vi "run.vi"(8 "error in (no error)":errorcluster, 11 "AutoExp in":refnum<class "AutoExp.lvclass">) -> (0 "error out":errorcluster, 3 "AutoExp out":refnum<class "AutoExp.lvclass">)   [LabVIEW 2018, in "AutoExp.lvclass"]
uses:
  AutoExp.lvclass
  AutoExp.lvclass/AutoExp.ctl
  State Machine/State Machine.lvclass
  Channel/Channel.lvclass
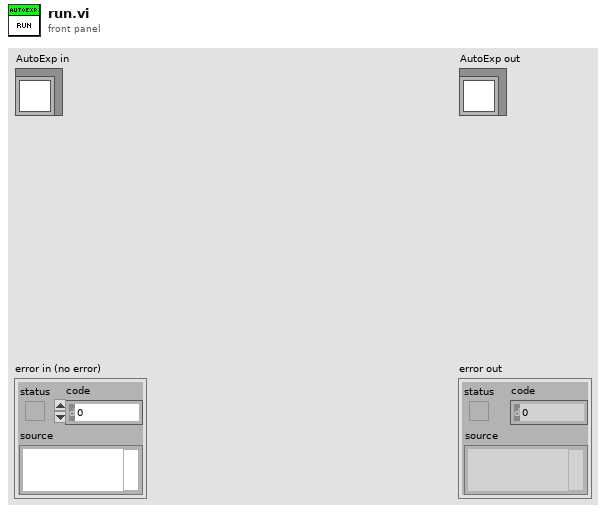
[diagram p1: front panel]
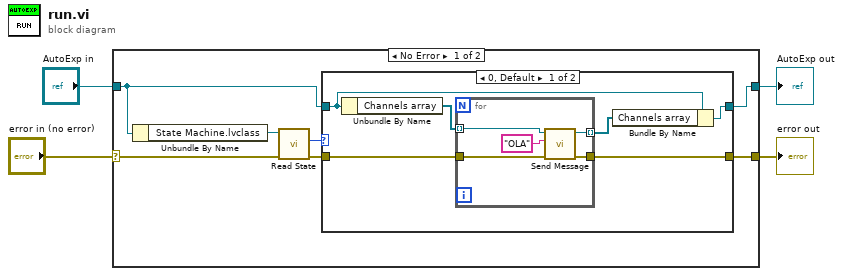
[diagram p0: block diagram]
diagram:
  n1 = case shown="No Error" "error in (no error)" {
    selector: "error in (no error)" -> [w11 w26]
    tunnel: [w7 w26] -> w3
    tunnel: [w5 w25] -> w1
    tunnel: "AutoExp in" -> [w6 w25]
    frame No Error {
      n2 = Unbundle By Name(w6) -> ("State Machine.lvclass"=w10:refnum<class "State Machine.lvclass">)
      n3 = call-dynamic "Read State.vi"("error in (no error)"=w11, "State Machine in"=w10) -> ("error out"=w8:errorcluster, "State"=w9:u16)  [unwired: 7 in, 1 out]
      n4 = case shown="0, Default" w9 {
        tunnel: w8 -> [w16 w23]
        tunnel: [w15 w23] -> w7
        tunnel: w6 -> [w14 w24]
        tunnel: [w12 w24] -> w5
        frame 0, Default {
          n5 = Unbundle By Name(w14) -> ("Channels array"=w17:refnum<class "Channel.lvclass">[])
          n6 = for {
            tunnel: w17 -> [w22] mode=indexing
            tunnel: w16 -> [w21]
            tunnel: [w20] -> w15
            tunnel: [w19] -> w13 mode=indexing
            n7 = call "Send Message.vi"("error in (no error)"=w21, "message"="OLA", "Channel in"=w22) -> ("error out"=w20:errorcluster, "Channel out"=w19:refnum<class "Channel.lvclass">)  [unwired: 7 in]
          }
          n8 = Bundle By Name(cluster=w14, "Channels array"=w13) -> (w12:refnum<class "AutoExp.lvclass">)
        }
        frame 1 {
        }
      }
    }
    frame Error {
    }
  }
  "error out" <- w3
  "AutoExp out" <- w1
